vi "Find Timeout.vi"(11 "Status":T1={"VI"={"error"={"status"=FALSE, "code"=0, "source"=""}, "isExiting?"=FALSE}, "UserLoggedIn?"=FALSE, "Processors"={"Averaging Type"=enum."Normal Average", "Roughness Processor"=refnum, "Objects"={"Video A"=refnum, "Video B"=refnum}, "Use Camera A?"=FALSE, "Use Camera B?"=FALSE}, "Playback"={"FPS"=10.0, "Playing?"=FALSE, "Playable?"=FALSE, "Image A"=refnum, "Image B"=refnum}, "Mouse Position A"=0.0, "Mouse Position B"=0.0}) -> (3 "Timeout":i32)   [LabVIEW 2018]
uses:
  Status STYP.ctl
  Video Processor/Video Processor.lvclass
  Roughness Averager/Roughness Averager.lvclass
  <vilib>/vision/Image Controls.llb/IMAQ Image.ctl
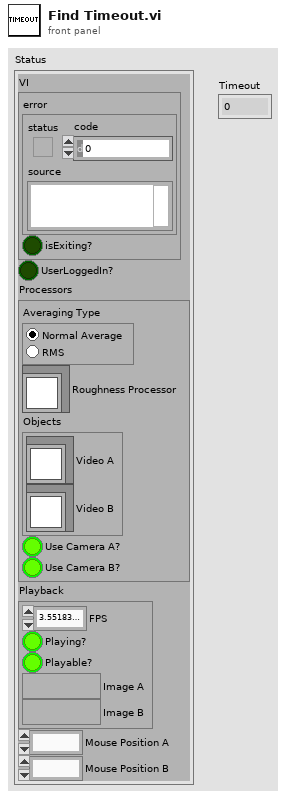
[diagram p1: front panel]
types:
  T1 = typedef "Status STYP.ctl" = cluster{"VI":cluster{"error":errorcluster, "isExiting?":bool}, "UserLoggedIn?":bool, "Processors":cluster{"Averaging Type":enum32{"Normal Average", "RMS"}, "Roughness Processor":refnum<class "Roughness Averager.lvclass">, "Objects":cluster{"Video A":refnum<class "Video Processor.lvclass">, "Video B":refnum<class "Video Processor.lvclass">}, "Use Camera A?":bool, "Use Camera B?":bool}, "Playback":cluster{"FPS":dbl, "Playing?":bool, "Playable?":bool, "Image A":T2, "Image B":T2}, "Mouse Position A":dbl, "Mouse Position B":dbl}
  T2 = typedef "IMAQ Image.ctl" = refnum<image>
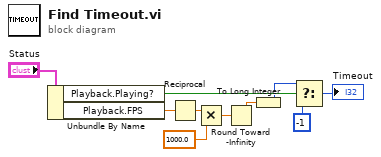
[diagram p0: block diagram]
diagram:
  n1 = Unbundle By Name("Status") -> ("Playback.Playing?"=w3:bool, "Playback.FPS"=w9:dbl)
  n2 = Reciprocal(x=w9) -> (1/x=w8:dbl)
  n3 = Multiply(x=w8, y=1000.0) -> (x*y=w6:dbl)
  n4 = Round Toward -Infinity(1:w6) -> (0:w4:dbl)
  n5 = To Long Integer(number=w4) -> (32bit integer=w2:i32)
  n6 = Select(t=w2, s=w3, f=-1 ("t")) -> (s? t:f=→"Timeout":i32)
